vi "response.To JSON Tree.vi"(8 "error in (no error)":errorcluster, 11 "Response in":refnum<class "Response.lvclass">) -> (0 "error out":errorcluster, 2 "JSON Value out":variant, 3 "Response out":refnum<class "Response.lvclass">)   [LabVIEW 2020, in "JSON-RPC Lib.lvlib" / "Response.lvclass"]
uses:
  Response.lvclass
  Response.lvclass/Response.ctl
  Variant Data Manipulation/Insert Element at Start.vi
  response.Has ID.vi
  response.Has Error.vi
  Variant Data Manipulation/Insert Element at End.vi
  error/error.lvclass
  id/id.lvclass
  result/result.lvclass
  Variant Data Manipulation/Variant Data Manipulation.lvlib
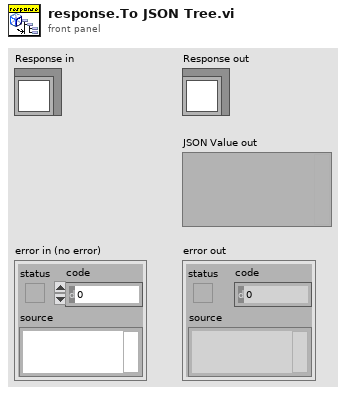
[diagram p1: front panel]
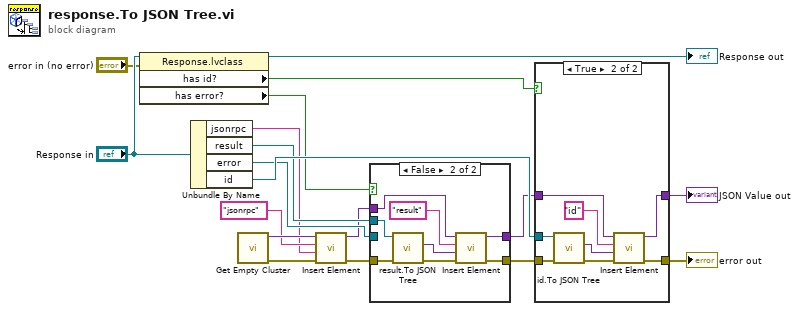
[diagram p0: block diagram]
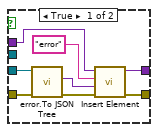
[diagram p2: hidden frame]
diagram:
  n1 = property class="Response.lvclass"(reference="Response in", error in="error in (no error)") -> (reference out=→"Response out":refnum<class "Response.lvclass">, "has id?"=w17:bool, "has error?"=w12:bool)  [unwired: 1 out]
  n2 = Unbundle By Name("Response in") -> ("jsonrpc"=w1:string, "result"=w14:refnum<class "result.lvclass">, "error"=w13:refnum<class "error.lvclass">, "id"=w16:refnum<class "id.lvclass">)
  n3 = call "Get Empty Cluster.vi"() -> ("error out"=w9:errorcluster, "Variant (Cluster) out"=w10:variant)  [unwired: 10 in]
  n4 = call-poly "Insert Element.vi"("error in (no error)"=w9, "element"=w1, "Name"="jsonrpc", "Variant (Cluster) in"=w10) -> ("error out"=w6:errorcluster, "Variant (Cluster) out"=w8:variant)  [unwired: 6 in]
  n5 = case shown="False" w12 {
    tunnel: w13 -> [w25 _]
    tunnel: w14 -> [_ w30]
    tunnel: w8 -> [w23 w32]
    tunnel: [w22 w31] -> w7
    tunnel: w6 -> [w21 w28]
    tunnel: [w19 w29] -> w5
    frame True {
      n6 = call "error.To JSON Tree.vi"("error in (no error)"=w21, "error in"=w25) -> ("error out"=w20:errorcluster, "JSON Value out"=w24:variant)  [unwired: 7 in, 1 out]
      n7 = call-poly "Insert Element.vi"("error in (no error)"=w20, "element"=w24, "Name"="error", "Cluster in"=w23) -> ("error out"=w19:errorcluster, "Cluster out"=w22:variant)  [unwired: 6 in]
    }
    frame False {
      n8 = call "result.To JSON Tree.vi"("error in (no error)"=w28, "result in"=w30) -> ("error out"=w27:errorcluster, "JSON Value out"=w33:variant)  [unwired: 7 in, 1 out]
      n9 = call-poly "Insert Element.vi"("error in (no error)"=w27, "element"=w33, "Name"="result", "Cluster in"=w32) -> ("error out"=w29:errorcluster, "Cluster out"=w31:variant)  [unwired: 6 in]
    }
  }
  n10 = case shown="True" w17 {
    tunnel: w16 -> [_ w44]
    tunnel: w7 -> [w35 w43]
    tunnel: w5 -> [w36 w40]
    tunnel: [w36 w38] -> w4
    tunnel: [w35 w37] -> w3
    frame False {
    }
    frame True {
      n11 = call "id.To JSON Tree.vi"("error in (no error)"=w40, "id in"=w44) -> ("error out"=w39:errorcluster, "JSON Value out"=w42:variant)  [unwired: 7 in, 1 out]
      n12 = call-poly "Insert Element.vi"("error in (no error)"=w39, "element"=w42, "Name"="id", "Cluster in"=w43) -> ("error out"=w38:errorcluster, "Cluster out"=w37:variant)  [unwired: 6 in]
    }
  }
  "error out" <- w4
  "JSON Value out" <- w3
